vi "Pre Launch Init.vi"(11 "UI Window in":refnum<class "UI Window.lvclass">) -> (0 "error out":errorcluster, 3 "UI Window out":refnum<class "UI Window.lvclass">)   [LabVIEW 2015, in "UI Window.lvlib" / "UI Window.lvclass"]
doc: "(<B>Filename</B>: Actor Framework.lvlib:Actor.lvclass:Pre Launch Init.vi)\n\nDefines behavior that occurs after the Launch Actor method is invoked but before the actor's Actor Core method begins running.\n\nThe Pre Launch Init method is guaranteed to finish before the Launch Actor method returns to its caller and before the actor itself receives any messages. Any references that the Pre Launch Init method obtains are guaranteed to have the same lifetime as the actor itself. Any errors that the Pre Launch Init method returns will abort the launch.\n\nBy default, this method does nothing. A descendant class may override it to define behavior."
uses:
  UI Window.lvclass
  <vilib>/ActorFramework/Actor/Actor.lvclass
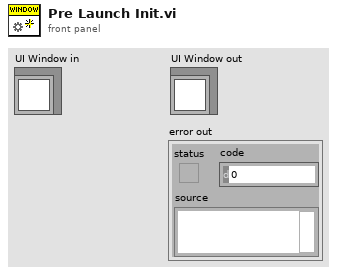
[diagram p1: front panel]
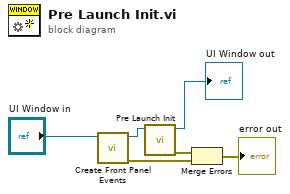
[diagram p0: block diagram]
diagram:
  n1 = call-dynamic "Create Front Panel Events.vi"("UI Window in"="UI Window in") -> ("error out"=w1:errorcluster, "UI Window out"=w2:refnum<class "UI Window.lvclass">)  [unwired: 9 in]
  n2 = call-parent "Pre Launch Init.vi"("Actor in"=w2) -> ("error out"=w3:errorcluster, "Actor out"=→"UI Window out":refnum<class "UI Window.lvclass">)  [unwired: 9 in]
  n3 = Merge Errors(w3, w1) -> (→"error out":errorcluster)
